vi "AD5933_ReadStatus (NI-845x I2C)(SubVI).vi"(7 "error in":errorcluster, 10 "NI-845x Config for I2C (in)":cluster{"i2c configuration":T1, "Refnum in":T2}) -> (0 "error out":errorcluster, 1 "Status Info":T4, 3 "NI-845x Config for I2C (out)":T3)   [LabVIEW 2017]
uses:
  <vilib>/ni845x/ni845x.llb/ni845xI2cConfiguration.ctl
  <vilib>/ni845x/ni845x.llb/ni845xControl.ctl
  TypeDefs/AD5933_CommandCodes.ctl
  TypeDefs/AD5933_Registers.ctl
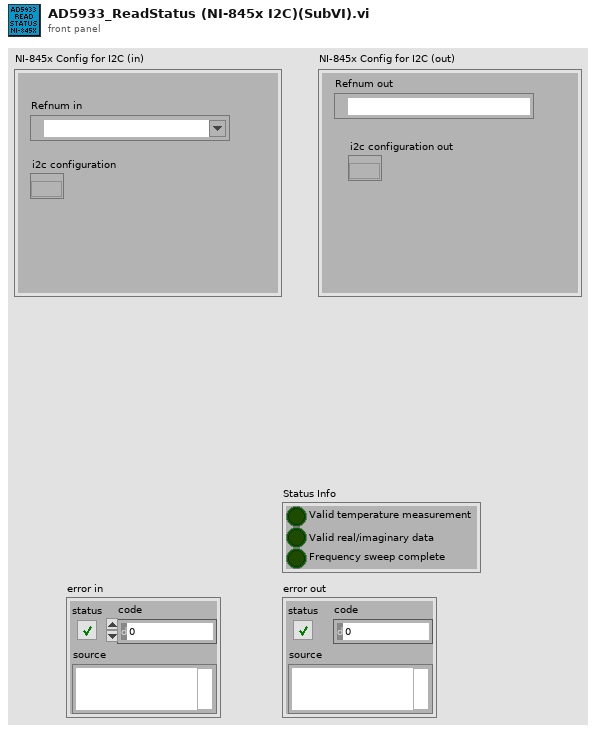
[diagram p1: front panel]
types:
  T1 = typedef "ni845xI2cConfiguration.ctl" = refnum<k20>
  T2 = typedef "ni845xControl.ctl" = refnum<k21>
  T3 = cluster{"i2c configuration out":T1, "Refnum out":T2}
  T4 = cluster{"Valid temperature measurement":bool, "Valid real/imaginary data":bool, "Frequency sweep complete":bool}
  T5 = typedef "AD5933_Registers.ctl" = u8
  T6 = typedef "AD5933_CommandCodes.ctl" = u8
  T7 = cluster{"Boolean array[0]":bool, "Boolean array[1]":bool, "Boolean array[2]":bool}
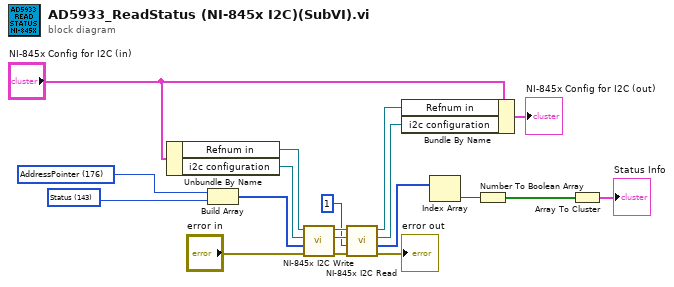
[diagram p0: block diagram]
diagram:
  w2 = T5 143 items=["Control_1"=128, "Control_0"=129, "StartFeq_2"=130, "StartFeq_1"=131, "StartFeq_0"=132, "FreqInc_2"=133, "FreqInc_1"=134, "FreqInc_0"=135, "NumOfInc_1"=136, "NumOfInc_0"=137, "NumOfSetCycl_1"=138, "NumOfSetCycl_0"=139, "Status"=143, "TempData_1"=146, "TempData_0"=147, "RealData_1"=148, "RealData_0"=149, "ImagData_1"=150, "ImagData_0"=151] ("Register")
  w3 = T6 176 items=["BlockWrite"=160, "BlockRead"=161, "AddressPointer"=176] ("CommandCodes")
  n1 = Unbundle By Name("NI-845x Config for I2C (in)") -> ("Refnum in"=w7:T2, "i2c configuration"=w8:T1)
  n2 = Build Array(w3, w2) -> (w16:T5[])
  n3 = call <vilib>:"NI-845x I2C Write.vi"("error in (no error)"="error in", "write data"=w16, "i2c configuration in"=w8, "device reference in"=w7) -> ("error out"=w15:errorcluster, "i2c configuration out"=w13:T1, "device reference out"=w12:T2)  [unwired: 5 in]
  n4 = call <vilib>:"NI-845x I2C Read.vi"("error in (no error)"=w15, "num bytes to read"=u32 1, "i2c configuration in"=w13, "device reference in"=w12) -> ("error out"=→"error out":errorcluster, "read data"=w17:u8[], "i2c configuration out"=w5:T1, "device reference out"=w6:T2)  [unwired: 4 in]
  n5 = Bundle By Name(cluster="NI-845x Config for I2C (in)", "Refnum in"=w6, "i2c configuration"=w5) -> (→"NI-845x Config for I2C (out)":cluster{"i2c configuration":T1, "Refnum in":T2})
  n6 = Index Array(array=w17) -> (element=w18:u8)  [unwired: 1 in]
  n7 = Number To Boolean Array(number=w18) -> (Boolean array=w1:bool[])
  n8 = Array To Cluster(array=w1) -> (cluster=→"Status Info":T7)
